vi "Function and Derivatives CG.vi"(9 "Parsed Formula":cluster{"table":i32[][], "result":dbl[]}, 10 "Variables":i32[](array[numeric])=[0, 0], 11 "X":dbl[](array[numeric]) format="%.2f") -> (2 "df/dX":dbl[](array[numeric]) format="%.2f", 3 "f(X)":dbl format="%.2f")   [LabVIEW 2017, in "NI_Gmath.lvlib"]
uses:
  NI_Gmath.lvlib
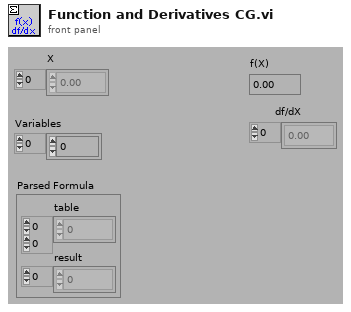
[diagram p1: front panel]
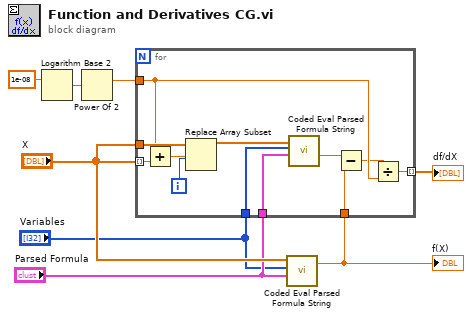
[diagram p0: block diagram]
diagram:
  n1 = Logarithm Base 2(1:1e-08) -> (0:w7:dbl)
  n2 = Power Of 2(x=w7) -> (2^x=w6:dbl)
  n3 = call "Coded Eval Parsed Formula String.vi"("Parsed Formula"="Parsed Formula", "Variables"="Variables", "X Values"="X") -> ("y value"=w5:dbl)  [unwired: 1 in, 1 out]
  "f(X)" <- w5
  n4 = for {
    tunnel: "X" -> [w20] mode=indexing
    tunnel: w6 -> [w14]
    tunnel: "X" -> [w19]
    tunnel: w5 -> [w15]
    tunnel: [w12] -> w4 mode=indexing
    tunnel: "Parsed Formula" -> [w10]
    tunnel: "Variables" -> [w9]
    i -> [w18]
    n5 = Add(x=w14, y=w20) -> (x+y=w17:dbl)
    n6 = Replace Array Subset(array=w19, new element=w17, index=w18) -> (w11:dbl[])
    n7 = call "Coded Eval Parsed Formula String.vi"("Parsed Formula"=w10, "Variables"=w9, "X Values"=w11) -> ("y value"=w16:dbl)  [unwired: 1 in, 1 out]
    n8 = Subtract(x=w16, y=w15) -> (x-y=w13:dbl)
    n9 = Divide(x=w13, y=w14) -> (x/y=w12:dbl)
  }
  "df/dX" <- w4
